vi "Discard.vi"(2 "count array":T1[](array[typedef]), 3 "% to discard":dbl) -> (16 "Array out":T1[](array[typedef]))   [LabVIEW 2013]
uses:
  _RTUtility_win.llb/NI Timestamp.ctl
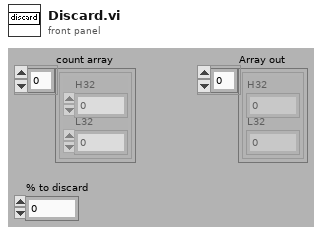
[diagram p1: front panel]
types:
  T1 = typedef "NI Timestamp.ctl" = cluster{"H32":u32, "L32":u32}
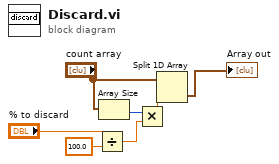
[diagram p0: block diagram]
diagram:
  n1 = Divide(x="% to discard", y=100.0) -> (x/y=w6:dbl)
  n2 = Array Size(array="count array") -> (size(s)=w1:i32)
  n3 = Multiply(x=w1, y=w6) -> (x*y=w3:dbl)
  n4 = Split 1D Array(array="count array", index=w3) -> (second subarray=→"Array out":T1[])  [unwired: 1 out]
